vi "initialInternakConf.vi"(8 "error in (no error)":errorcluster, 11 "ElectrometerInternalConfiguration in":refnum<class "ElectrometerInternalConfiguration.lvclass">) -> (0 "error out":errorcluster, 3 "ElectrometerInternalConfiguration out":refnum<class "ElectrometerInternalConfiguration.lvclass">)   [LabVIEW 2016, in "ElectrometerInternalConfiguration.lvclass"]
uses:
  ElectrometerInternalConfiguration.lvclass
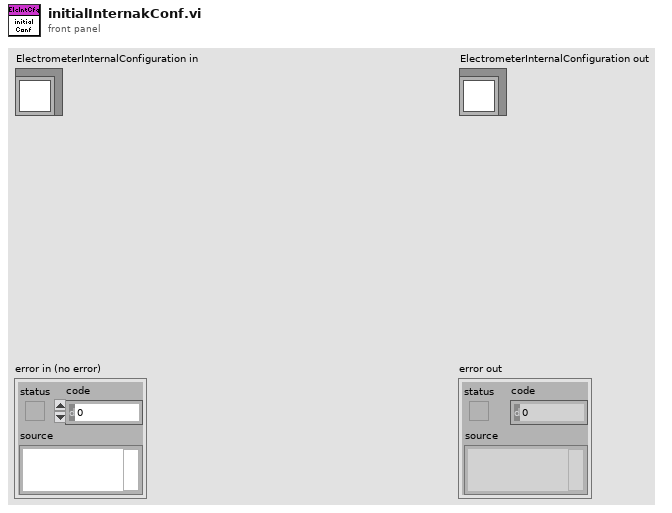
[diagram p1: front panel]
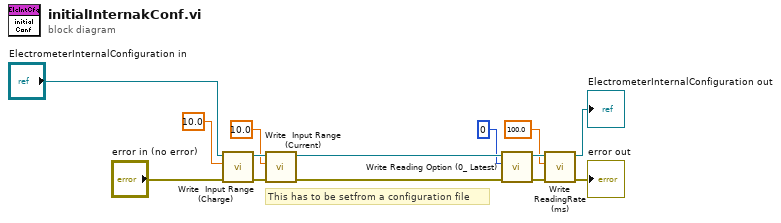
[diagram p0: block diagram]
diagram:
  # "This has to be setfrom a configuration file"
  n1 = call-dynamic "Write  Input Range (Charge).vi"("error in (no error)"="error in (no error)", "Input Range (Charge)"=10.0, "ElectrometerInternalConfiguration in"="ElectrometerInternalConfiguration in") -> ("error out"=w8:errorcluster, "ElectrometerInternalConfiguration out"=w13:refnum<class "ElectrometerInternalConfiguration.lvclass">)  [unwired: 7 in]
  n2 = call-dynamic "Write  Input Range (Current).vi"("error in (no error)"=w8, "Input Range (Current)"=10.0, "ElectrometerInternalConfiguration in"=w13) -> ("error out"=w7:errorcluster, "ElectrometerInternalConfiguration out"=w12:refnum<class "ElectrometerInternalConfiguration.lvclass">)  [unwired: 7 in]
  n3 = call-dynamic "Write Reading Option (0_ Latest).vi"("error in (no error)"=w7, "Reading Option (0: Latest)"=0, "ElectrometerInternalConfiguration in"=w12) -> ("error out"=w6:errorcluster, "ElectrometerInternalConfiguration out"=w11:refnum<class "ElectrometerInternalConfiguration.lvclass">)  [unwired: 7 in]
  n4 = call-dynamic "Write ReadingRate (ms).vi"("error in (no error)"=w6, "ReadingRate (ms)"=100.0, "ElectrometerInternalConfiguration in"=w11) -> ("error out"=→"error out":errorcluster, "ElectrometerInternalConfiguration out"=→"ElectrometerInternalConfiguration out":refnum<class "ElectrometerInternalConfiguration.lvclass">)  [unwired: 7 in]
